vi "S2DS_New header.vi"(2 "Complete channel name info":T1={"WCl names with units"=[], "RC  names with units"=[], "DC  names with units"=[""], "AC names with units"=[], "Indicator captions"=[], "Graph channels"=[], "Channel numbers"=[], "User info"=""}) -> (0 "Header (out)":string)   [LabVIEW 2025]
uses:
  TYPE DEFS/S2DS_Display info.ctl
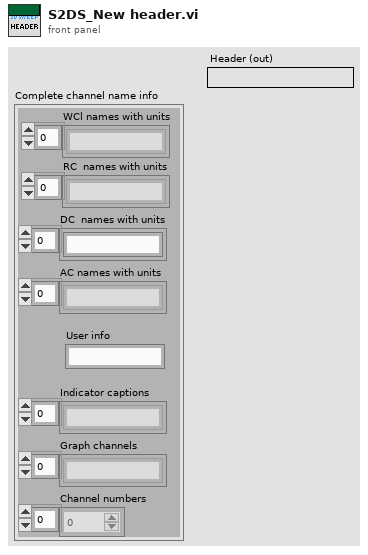
[diagram p1: front panel]
types:
  T1 = typedef "S2DS_Display info.ctl" = cluster{"WCl names with units":string[], "RC  names with units":string[], "DC  names with units":string[], "AC names with units":string[], "Indicator captions":string[], "Graph channels":string[], "Channel numbers":i32[], "User info":string}
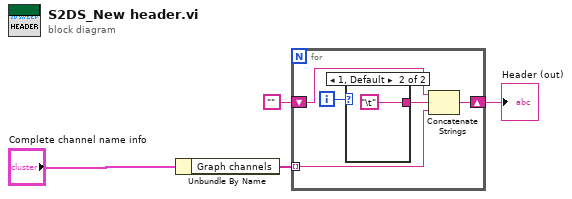
[diagram p0: block diagram]
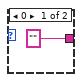
[diagram p2: hidden frame]
diagram:
  n1 = Unbundle By Name("Complete channel name info") -> ("Graph channels"=w2:string[])
  n2 = for {
    tunnel: w2 -> [w8] mode=indexing
    shift-right: [w9] -> w1
    shift-left: "" -> [w6]
    i -> [w7]
    n3 = case shown="1, Default" w7 {
      tunnel: ["" "\t"] -> w5
      frame 0 {
      }
      frame 1, Default {
      }
    }
    n4 = Concatenate Strings(w6, w5, w8) -> (w9:string)
  }
  "Header (out)" <- w1
